vi "Degrees to Radians (Array SGL).vi"(3 "angles (deg)":sgl[](array[numeric]) caption="角（角度）") -> (1 "angles (rad)":sgl[](array[numeric]) caption="角（弧度）")   [LabVIEW 2011, in "NI_AngleManipulation.lvlib"]
doc: "Converts a 1D array of angles from degrees to radians."
uses:
  <vilib>/Utility/AngleManip/NI_AngleManipulation.lvlib
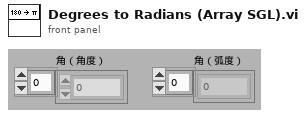
[diagram p1: front panel]
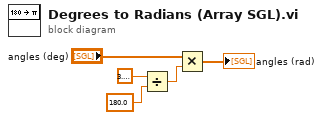
[diagram p0: block diagram]
diagram:
  n1 = Divide(x=sgl 3.1415927, y=sgl 180.0) -> (x/y=w3:sgl)
  n2 = Multiply(x="angles (deg)", y=w3) -> (x*y=→"angles (rad)":sgl[])
